vi "UserVars-Parse Vector Expression.vi"(0 "Expression In":string, 7 "first var":i32, 11 "error in (no error)":errorcluster) -> (4 "Expression Out":string, 8 "values":dbl[][](array[numeric]), 10 "variables":string[](array[string]), 15 "error out":errorcluster)   [LabVIEW 2020]
uses:
  <vilib>/regexp/Match Regular Expression.xnode
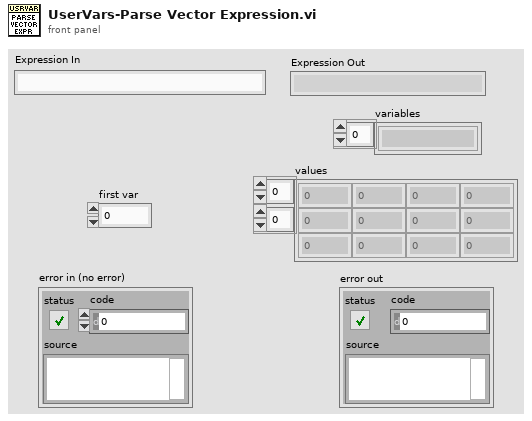
[diagram p1: front panel]
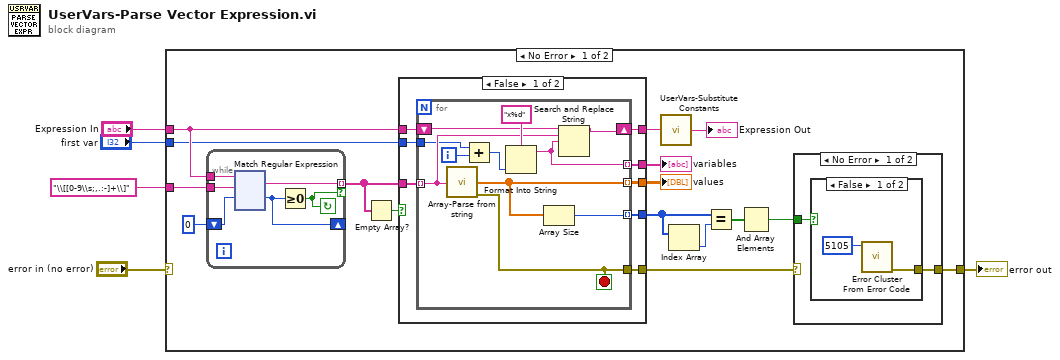
[diagram p0: block diagram]
diagram:
  n1 = case shown="No Error" "error in (no error)" {
    selector: "error in (no error)" -> [_ w167]
    tunnel: "\\[[0-9\\s;,.:-]+\\]" ("regular expression") -> [w21 _]
    tunnel: "Expression In" -> [w18 _]
    tunnel: [w12 w167] -> w3
    tunnel: "first var" -> [w6 _]
    frame No Error {
      n2 = while {
        tunnel: w18 -> [w52]
        tunnel: w21 -> [w51]
        shift-right: [w49] -> _
        shift-left: 0 -> [w50]
        tunnel: [w48] -> w10 mode=indexing if=w47
        stop <- w47 continue-if-true
        n3 = xnode "Match Regular Expression"("input string"=w52, "regular expression"=w51, "offset (0)"=w50) -> ("whole match"=w48:string, "offset past match"=w49:i32)  [unwired: 3 in, 3 out]
        n4 = Greater Or Equal To 0?(x=w49) -> (x >= 0?=w47:bool)
      }
      n5 = Empty Array?(array=w10) -> (empty?=w9:bool)
      n6 = case shown="False" w9 {
        tunnel: w10 -> [w29 _]
        tunnel: [w28 _] -> w19
        tunnel: w18 -> [w27 w41]
        tunnel: [w26 _] -> w17
        tunnel: [w25 _] -> w14
        tunnel: [w24 _] -> w11
        tunnel: [w23 w41] -> w8
        tunnel: w6 -> [w22 _]
        frame False {
          n7 = for {
            tunnel: w29 -> [w37] mode=indexing
            tunnel: [w36] -> w28 mode=indexing
            shift-right: [w38] -> w23
            shift-left: w27 -> [w39]
            tunnel: [w35] -> w26 mode=indexing
            tunnel: [w34] -> w25
            tunnel: [w33] -> w24 mode=indexing
            tunnel: w22 -> [w31]
            i -> [w32]
            stop <- w34 stop-if-true
            n8 = call "Array-Parse from string.vi"("String"=w37) -> ("Array"=w36:dbl[], "error out"=w34:errorcluster)  [unwired: 13 in]
            n9 = Add(x=w31, y=w32) -> (x+y=w30:i32)
            n10 = Format Into String(format string="x%d", w30) -> (resulting string=w33:string)  [unwired: 2 in, 1 out]
            n11 = Array Size(array=w36) -> (size(s)=w35:i32)
            n12 = Search and Replace String(input string=w39, search string=w37, replace string=w33) -> (result string=w38:string)  [unwired: 5 in, 3 out]
          }
        }
        frame True {
        }
      }
      "values" <- w19
      "variables" <- w11
      n13 = call "UserVars-Substitute Constants.vi"("Expression In"=w8) -> ("Expression Out"=→"Expression Out":string)  [unwired: 14 in]
      n14 = Index Array(array=w17) -> (element=w16:i32)  [unwired: 1 in]
      n15 = Equal?(x=w17, y=w16) -> (x = y?=w15:bool[])
      n16 = And Array Elements(Boolean array=w15) -> (logical AND=w13:bool)
      n17 = case shown="No Error" w14 {
        selector: w14 -> [_ w46]
        tunnel: w13 -> [w43 _]
        tunnel: [w42 w46] -> w12
        frame No Error {
          n18 = case shown="False" w43 {
            tunnel: [w44 _] -> w42
            frame False {
              n19 = call <vilib>:"Error Cluster From Error Code.vi"("error code (0)"=5105) -> ("error out"=w44:errorcluster)  [unwired: 8 in]
            }
            frame True {
            }
          }
        }
        frame Error {
        }
      }
    }
    frame Error {
    }
  }
  "error out" <- w3
